vi "未命名 1.vi"() -> ()   [LabVIEW 2012]
uses:
  <vilib>/Instr/_visa.llb/VISA Configure Serial Port (Instr).vi
panel:
  out "读取缓冲区":string
  in  "写入缓冲区":string
  in  "VISA resource name":refnum<visa-resource-name> caption="VISA资源名称"
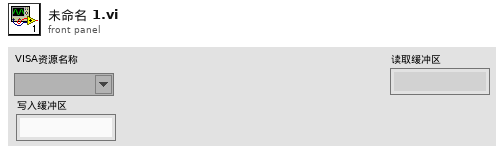
[diagram p1: front panel]
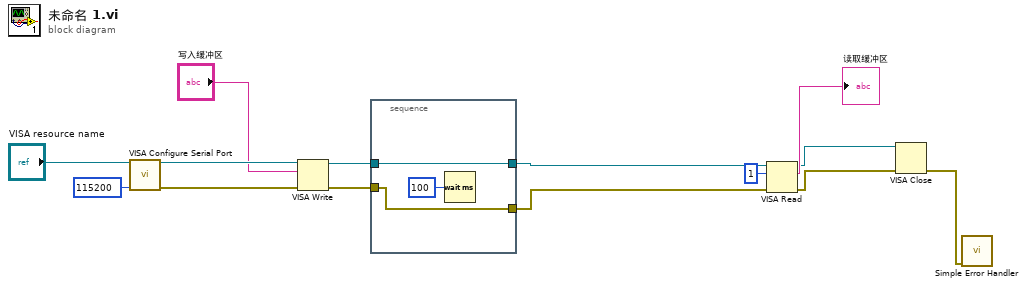
[diagram p0: block diagram]
diagram:
  n1 = call-poly "VISA Configure Serial Port"("VISA resource name"="VISA resource name", "baud rate (9600)"=u32 115200) -> ("VISA resource name out"=w13:refnum<visa-resource-name>, "error out"=w12:errorcluster)  [unwired: 12 in]
  n2 = VISA Write(VISA resource name=w13, write buffer="写入缓冲区", error in (no error)=w12) -> (VISA resource name out=w10:refnum<visa-resource-name>, error out=w9:errorcluster)  [unwired: 1 out]
  n3 = stacked-sequence {
    tunnel: w10 -> [w16]
    tunnel: w9 -> [w15]
    tunnel: [w16] -> w8
    tunnel: [w15] -> w7
    frame #0 {
      n4 = Wait (ms)(milliseconds to wait=u32 100 ("等待时间（毫秒）")) -> ()  [unwired: 1 out]
    }
  }
  n5 = VISA Read(VISA resource name=w8, byte count=u32 1 ("字节总数"), error in (no error)=w7) -> (VISA resource name out=w5:refnum<visa-resource-name>, read buffer=→"读取缓冲区":string, error out=w4:errorcluster)  [unwired: 1 out]
  n6 = VISA Close(VISA resource name=w5, error in (no error)=w4) -> (error out=w2:errorcluster)
  n7 = call <vilib>:"Simple Error Handler.vi"("error in (no error)"=w2) -> ()  [unwired: 4 in, 5 out]
